vi "WSVCAP SHL FPGA LL RFFE Read Data.vi"(11 "error in (no error)":errorcluster, 12 "Socket Mask":u64) -> (4 "Word Out (1-Bit for Each Channel)":u64, 15 "error out":errorcluster)   [LabVIEW 2012]
uses:
  <vilib>/rvi/eio/common/nirviEmuTemplateMethod_errors.vi
  <vilib>/eio/EIONode/EIONode.xnode
  WSVCAP SHL FPGA LL RFFE Debug Global.vi
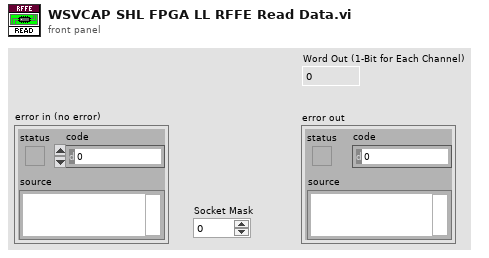
[diagram p1: front panel]
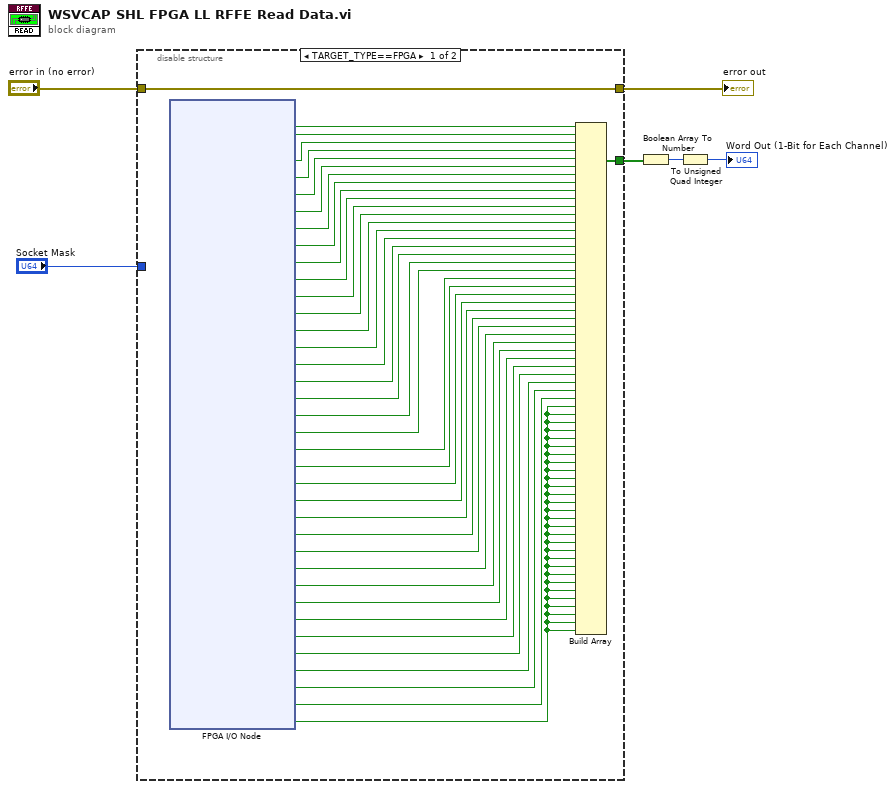
[diagram p0: block diagram]
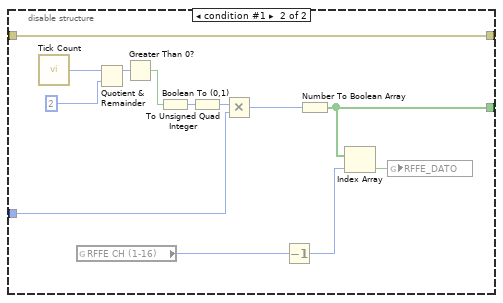
[diagram p2: hidden frame]
diagram:
  n1 = disable-structure shown="TARGET_TYPE==FPGA" {
    disable-tunnel: [w28 w47] -> w2
    disable-tunnel: [w27 w54] -> w6
    disable-tunnel: "error in (no error)" -> [w27 w54]
    disable-tunnel: "Socket Mask" -> [_ w51]
    frame condition #0 (active) {
      n2 = xnode "FPGA I/O Node"() -> ("RFFE_DATO_S1"=w29:bool, "RFFE_DATO_S2"=w44:bool, "RFFE_DATO_S3"=w43:bool, "RFFE_DATO_S4"=w42:bool, "RFFE_DATO_S5"=w41:bool, "RFFE_DATO_S6"=w40:bool, "RFFE_DATO_S7"=w39:bool, "RFFE_DATO_S8"=w38:bool, "RFFE_DATO_S9"=w37:bool, "RFFE_DATO_S10"=w36:bool, "RFFE_DATO_S11"=w35:bool, "RFFE_DATO_S12"=w34:bool, "RFFE_DATO_S13"=w33:bool, "RFFE_DATO_S14"=w32:bool, "RFFE_DATO_S15"=w31:bool, "RFFE_DATO_S16"=w30:bool, "RFFE_DATO_S17"=w26:bool, "RFFE_DATO_S18"=w25:bool, "RFFE_DATO_S19"=w24:bool, "RFFE_DATO_S20"=w23:bool, "RFFE_DATO_S21"=w22:bool, "RFFE_DATO_S22"=w21:bool, "RFFE_DATO_S23"=w20:bool, "RFFE_DATO_S24"=w19:bool, "RFFE_DATO_S25"=w18:bool, "RFFE_DATO_S26"=w17:bool, "RFFE_DATO_S27"=w16:bool, "RFFE_DATO_S28"=w15:bool, "RFFE_DATO_S29"=w14:bool, "RFFE_DATO_S30"=w13:bool, "RFFE_DATO_S31"=w12:bool, "RFFE_DATO_S32"=w11:bool, "RFFE_DATO_S33"=w10:bool, "RFFE_DATO_S34"=w9:bool, "RFFE_DATO_S35"=w8:bool, "RFFE_DATO_S36"=w7:bool)  [unwired: 36 in, 36 out]
      n3 = Build Array(w29, w44, w43, w42, w41, w40, w39, w38, w37, w36, w35, w34, w33, w32, w31, w30, w26, w25, w24, w23, w22, w21, w20, w19, w18, w17, w16, w15, w14, w13, w12, w11, w10, w9, w8, w7, w7, w7, w7, w7, w7, w7, w7, w7, w7, w7, w7, w7, w7, w7, w7, w7, w7, w7, w7, w7, w7, w7, w7, w7, w7, w7, w7, w7) -> (w28:bool[])
    }
    frame condition #1 {
      n4 = call "Tick Count"() -> ("Tick Count(Ticks)"=w57:u32)
      n5 = global read "WSVCAP SHL FPGA LL RFFE Debug Global.vi" "RFFE CH (1-16)"() -> (w49:i32)
      n6 = Quotient & Remainder(x=w57, y=u32 2) -> (x-y*floor(x/y)=w56:u32)  [unwired: 1 out]
      n7 = Greater Than 0?(x=w56) -> (x > 0?=w45:bool)
      n8 = Boolean To (0,1)(Boolean=w45) -> (0, 1=w53:i16)
      n9 = To Unsigned Quad Integer(1:w53) -> (0:w52:u64)
      n10 = Multiply(x=w52, y=w51) -> (x*y=w50:u64)
      n11 = Decrement(x=w49) -> (x-1=w46:i32)
      n12 = Number To Boolean Array(number=w50) -> (Boolean array=w47:bool[])
      n13 = Index Array(array=w47, index=w46) -> (element=w48:bool)
      n14 = global write "WSVCAP SHL FPGA LL RFFE Debug Global.vi" "RFFE_DATO"(w48) -> ()
    }
  }
  "error out" <- w6
  n15 = Boolean Array To Number(Boolean array=w2) -> (number=w3:u64)
  n16 = To Unsigned Quad Integer(1:w3) -> (0:→"Word Out (1-Bit for Each Channel)":u64)
